vi "CDW_SpecPage.vi"(10 "Spec Page Interface":T2, 11 "MetaDataObj in":refnum<class "MetaDataObj.lvclass">) -> (3 "MetaDataObj out":refnum<class "MetaDataObj.lvclass">)   [LabVIEW 2023, in "NIVS_Consolidated_CDW_MetaDataObj.lvclass"]
uses:
  NIVS_Consolidated_CDW_MetaDataObj.lvclass
  <resource>/dialog/NewProjectWizard/Spec Page Interface.ctl
  <resource>/dialog/NewProjectWizard/MetaDataObj/MetaDataObj.lvclass
  C:/Program Files/National Instruments/LabVIEW 2024/resource/dialog/NewProjectWizard/MetaDataObj/MetaDataObj.lvclass
  Template Classes/NIVS_Asynchronous/NIVS_Asynchronous.lvclass
  C:/dev/Karthick/FPGA Addons Packages/niveristand-custom-device-wizard/ProjectTemplate/Source/NI VeriStand/Custom Device/Template Classes/NIVS_CD Template/NIVS_CD Template.lvclass
  Template Classes/NIVS_Inline HW Interface (Inline-Async)/NIVS_Inline HW Interface (Inline-Async).lvclass
  Template Classes/NIVS_Inline HW Interface/NIVS_Inline HW Interface.lvclass
  Template Classes/NIVS_PPL_Inline HW Interface (Inline-Async)/NIVS_PPL_Inline HW Interface (Inline-Async).lvclass
  C:/dev/Karthick/FPGA Addons Packages/niveristand-custom-device-wizard/ProjectTemplate/Source/NI VeriStand/Custom Device/Template Classes/NIVS_PPLCD Template/NIVS_PPLCD Template.lvclass
  Template Classes/NIVS_PPL_Inline HW Interface/NIVS_PPL_Inline HW Interface.lvclass
  Template Classes/NIVS_Inline Model Interface/NIVS_Inline Model Interface.lvclass
  Template Classes/NIVS_Inline Timing and Sync/NIVS_Inline Timing and Sync.lvclass
  Template Classes/NIVS_Asynchronous Timing and Sync/NIVS_Asynchronous Timing and Sync.lvclass
  Template Classes/NIVS_CD Template/NIVS_CD Template.lvclass/NIVS_CD Template.ctl
  NIVS_Consolidated_CDW_MetaDataObj.lvclass/NIVS_Consolidated_CDW_MetaDataObj.ctl
  <resource>/dialog/NewProjectWizard/MetaDataObj/MetaDataObj.lvclass/MetaDataObj.ctl
  Execution Mode.ctl
  Template Classes/NIVS_CD Template/Write Max Instances.vi
  Template Classes/NIVS_CD Template/Write Extra Page Names.vi
  Template Classes/NIVS_CD Template/Write Submenu.vi
  Template Classes/NIVS_CD Template/Write Parent Menu.vi
  Template Classes/NIVS_CD Template/Write Support Runtime Configuration.vi
  <resource>/dialog/NewProjectWizard/MetaDataObj/Accessors/Write Project Name.vi
  <resource>/dialog/NewProjectWizard/MetaDataObj/Accessors/Write Project Root.vi
  Template Classes/NIVS_PPLCD Template/NIVS_PPLCD Template.lvclass
  Template Classes/NIVS_CD Template/NIVS_CD Template.lvclass
panel:
  in  "PPL Build":bool
  in  "Inline-Async":bool=TRUE
  in  "Custom Device Execution Mode":T1(ring)=enum."Inline HW Interface"
  in  "Custom Device Name":string
  in  "Project Root":path
  in  "Support Runtime Configuration":bool
  in  "Maximum Custom Device Instances":i32=1 min=-1 max=2474 step=1
  in  "Insert Custom Device in submenu":bool
  in  "Parent Menu Name":string
  in  "Custom Device Extra Page Names":string[](array[string])
  # "Advanced Options"
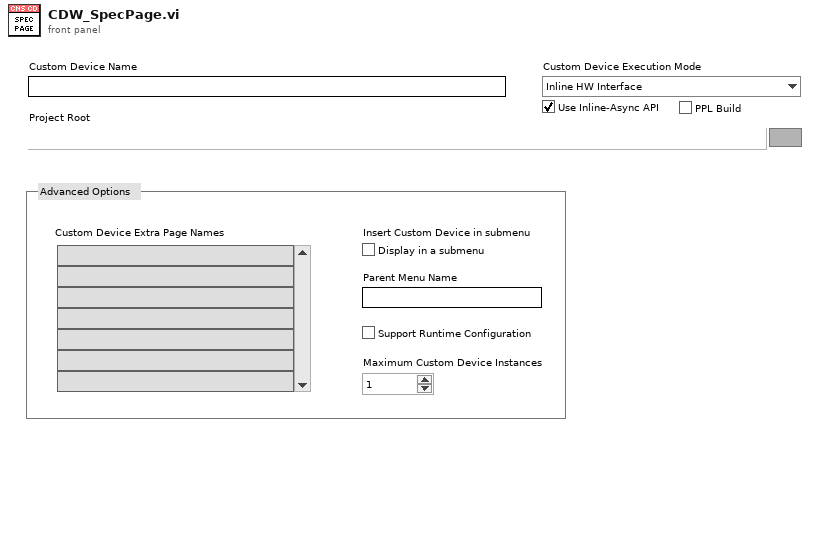
[diagram p1: front panel]
types:
  T1 = enum16{"Asynchronous", "Inline HW Interface", "Inline Model Interface", "Inline Timing and Sync", "Asynchronous Timing and Sync"}
  T2 = typedef "Spec Page Interface.ctl" = cluster{"\"Tab Forward To\" Refnum":refnum<vi>, "\"Tab Backward To\" Refnum":refnum<vi>, "Errors":refnum<user-event>, "Quit":refnum<user-event>}
  T3 = enum8{"Enabled", "Disabled", "Disabled and Grayed Out"}
  T4 = typedef "NIVS_Consolidated_CDW_MetaDataObj.lvclass/Execution Mode.ctl" = enum16{"Asynchronous", "Inline HW Interface", "Inline Model Interface", "Inline Timing and Sync", "Asynchronous Timing and Sync"}
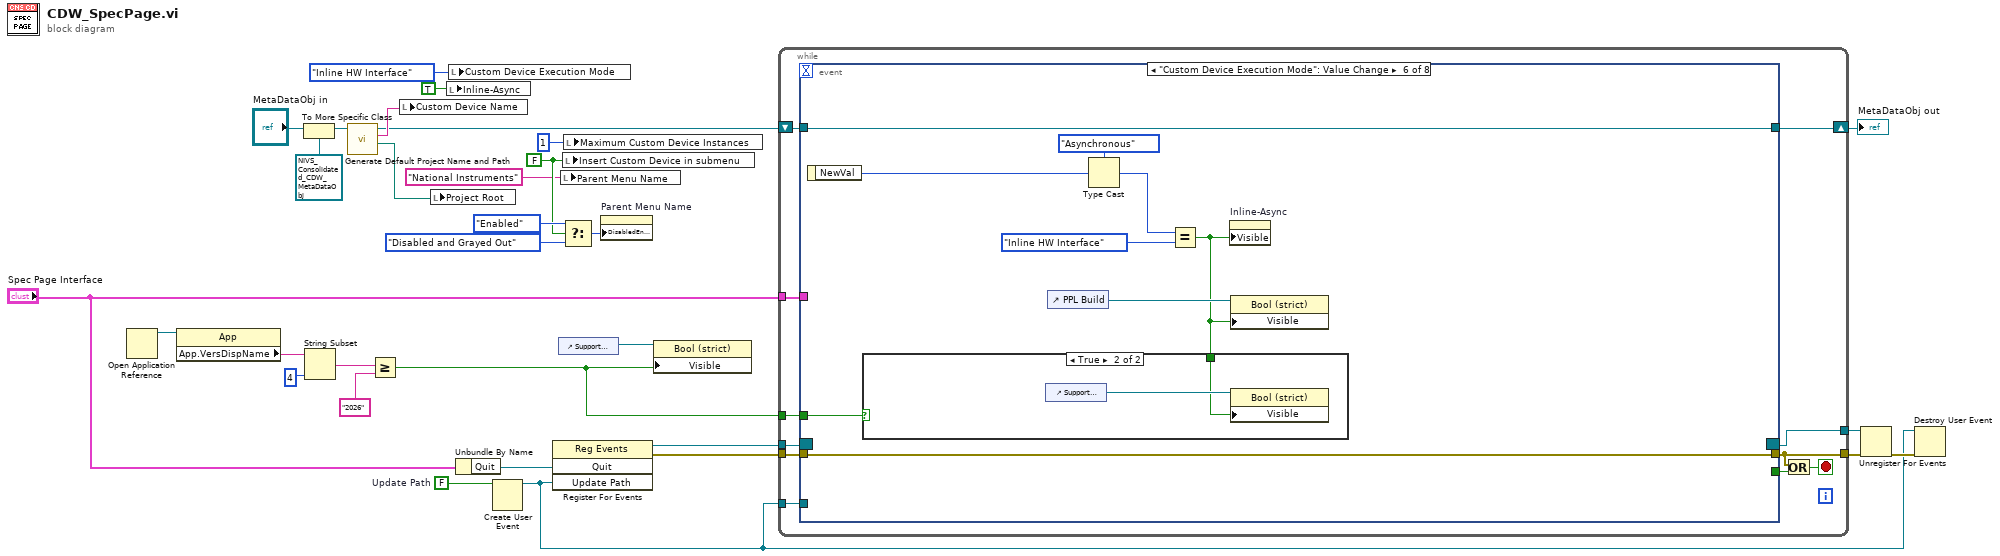
[diagram p0: block diagram]
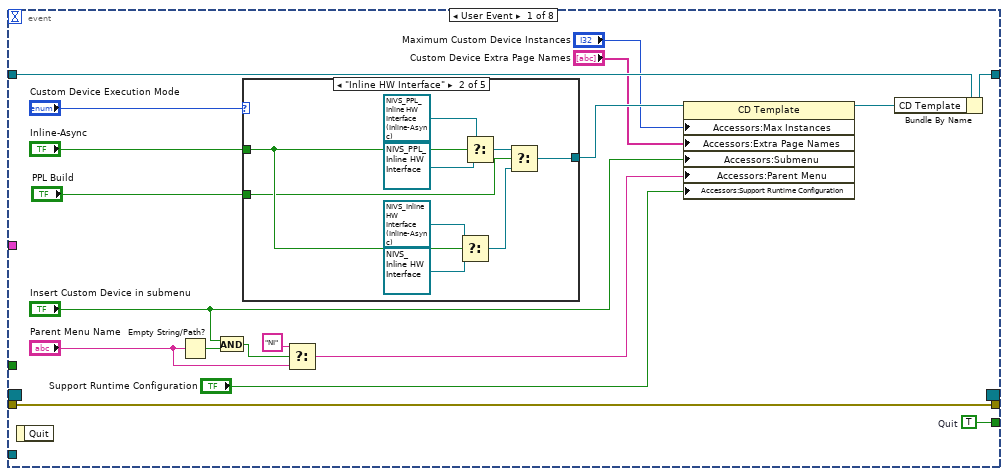
[diagram p2: hidden frame]
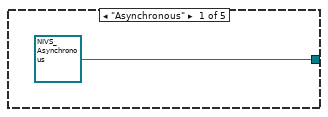
[diagram p3: hidden frame]
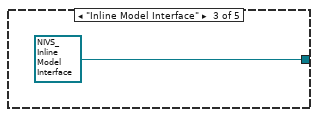
[diagram p4: hidden frame]
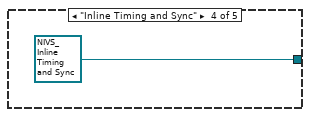
[diagram p5: hidden frame]
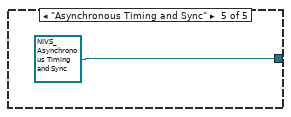
[diagram p6: hidden frame]
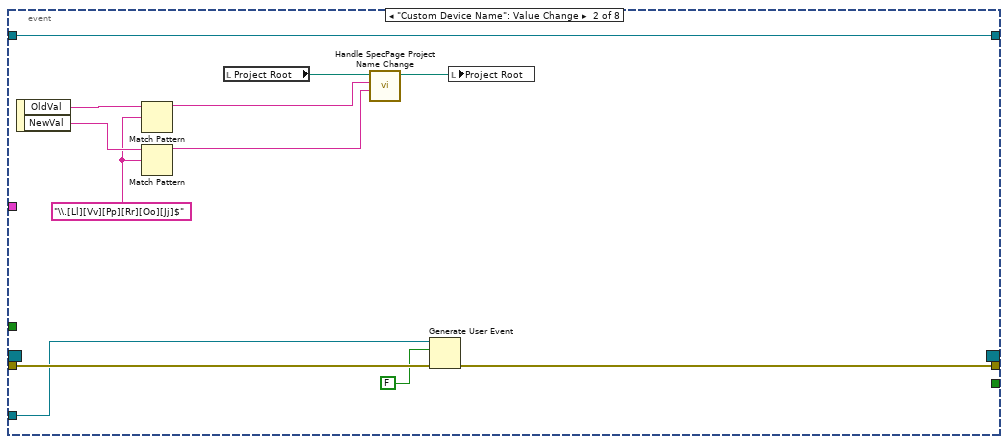
[diagram p7: hidden frame]
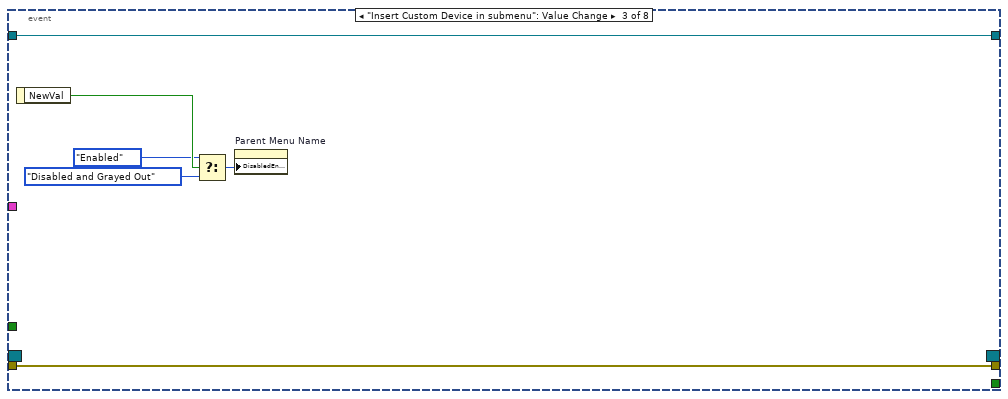
[diagram p8: hidden frame]
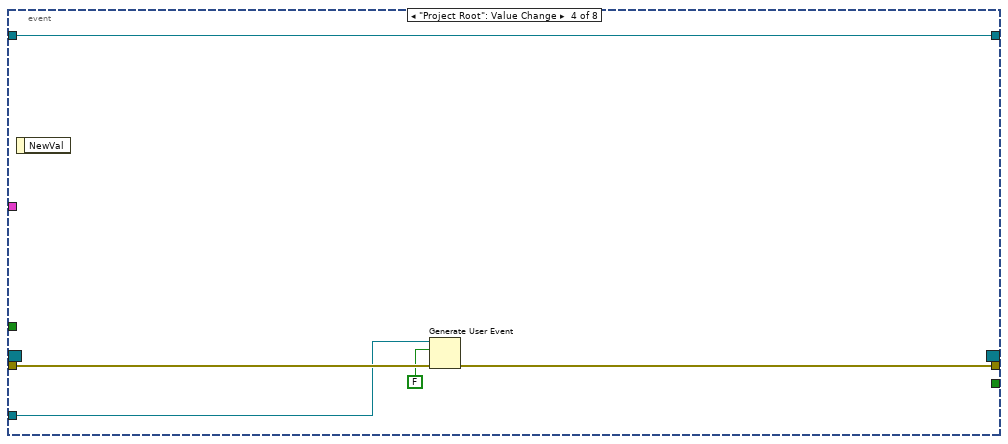
[diagram p9: hidden frame]
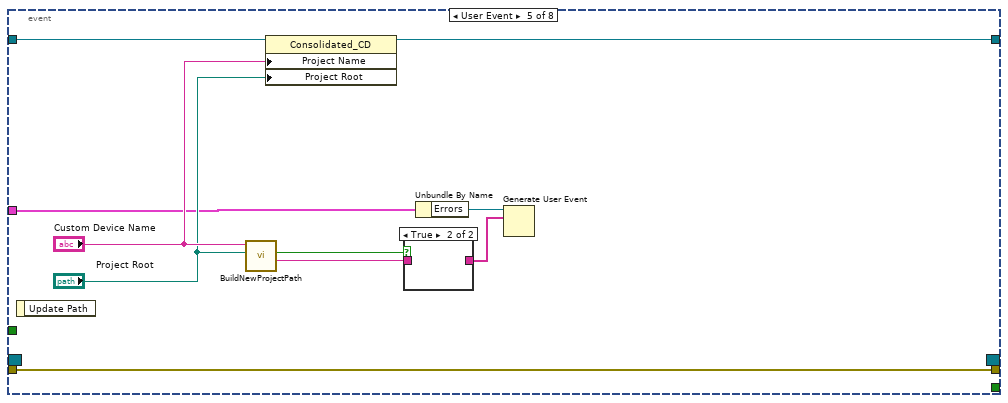
[diagram p10: hidden frame]
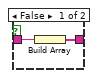
[diagram p11: hidden frame]
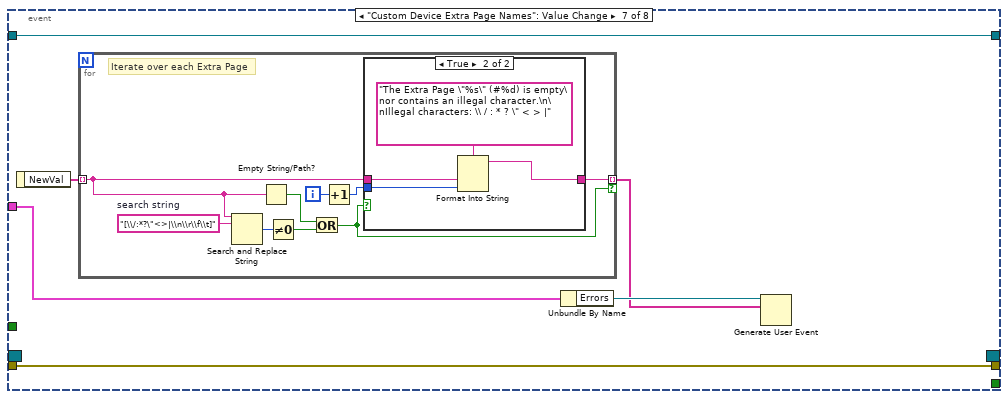
[diagram p13: hidden frame]
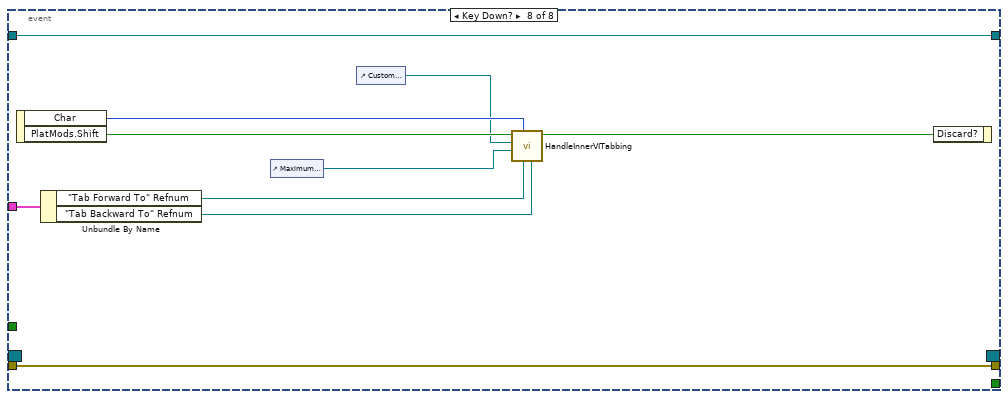
[diagram p15: hidden frame]
diagram:
  w12 = FALSE
  w15 = FALSE  # Update Path
  n1 = Open Application Reference() -> (3:w7:refnum<vi>)  [unwired: 4 in, 1 out]
  n2 = property class="App"(reference=w7) -> ("App.VersDispName"=w6:string)  [unwired: 1 in, 2 out]
  n3 = To More Specific Class(target class=refnum<class "NIVS_Consolidated_CDW_MetaDataObj.lvclass"> refnum ("Consolidated"), reference="MetaDataObj in") -> (specific class reference=w18:refnum<class "NIVS_Consolidated_CDW_MetaDataObj.lvclass">)  [unwired: 1 in, 1 out]
  n4 = String Subset(string=w6, length (rest)=4 ("length (rest)")) -> (substring=w5:string)  [unwired: 1 in]
  n5 = call <resource>:"Generate Default Project Name and Path.vi"("DNL_MetaDataObj in"=w18) -> ("Project Root"=w16:path, "Project Name"=w21:string, "DNL_MetaDataObj out"=w17:refnum<class "NIVS_Consolidated_CDW_MetaDataObj.lvclass">)  [unwired: 8 in]
  n6 = Greater Or Equal?(x=w5, y="2026") -> (x >= y?=w1:bool)
  n7 = local write "Custom Device Name"(w21) -> ()
  n8 = local write "Project Root"(w16) -> ()
  n9 = local write "Inline-Async"(TRUE ("Inline-Async")) -> ()
  n10 = local write "Custom Device Execution Mode"(T1."Inline HW Interface" ("Custom Device Execution Mode")) -> ()
  n11 = Unbundle By Name("Spec Page Interface") -> ("Quit"=w31:refnum<user-event>)
  n12 = Create User Event(user event datatype=w15) -> (user event=w13:refnum<user-event>)  [unwired: 1 in, 1 out]
  n13 = register-events(w31, w13) -> (reference out=w30:refnum<event-registration>, error out=w26:errorcluster)  [unwired: 2 in]
  n14 = control-ref of="Support Runtime Configuration"() -> (w2:refnum<vi>)
  n15 = local write "Parent Menu Name"("National Instruments") -> ()
  n16 = local write "Insert Custom Device in submenu"(w12) -> ()
  n17 = Select(t=T3."Enabled" ("Disabled"), s=w12, f=T3."Disabled and Grayed Out") -> (s? t:f=w24:T3)
  n18 = local write "Maximum Custom Device Instances"(u32 1 ("Maximum Custom Device Instances")) -> ()
  n19 = property on="Parent Menu Name" class="Str"("DisabledEnum"=w24) -> ()  [unwired: 2 in, 2 out]
  n20 = property class="Bool (strict)"(reference=w2, "Visible"=w1) -> ()  [unwired: 1 in, 2 out]
  n21 = while {
    tunnel: "Spec Page Interface" -> [w40]
    shift-right: [w39] -> w27
    shift-left: w17 -> [w38]
    tunnel: w30 -> [w42]
    tunnel: w26 -> [w41]
    tunnel: [w35] -> w28
    tunnel: [w34] -> w20
    tunnel: w13 -> [w33]
    tunnel: w1 -> [w32]
    stop <- w37 stop-if-true
    n22 = event shown="[5] \"Custom Device Execution Mode\": Value Change" {
      selector: w42 -> [_ _ _ _ _ _ _ _]
      dyn-events: [_ _ _ _ _ _ _ _] -> w34
      timeout: _ -> [_ _ _ _ _ _ _ _]
      tunnel: w40 -> [_ _ _ _ w101 _ w121 w144]
      tunnel: [w60 _ _ _ _ _ _ _] -> w36
      tunnel: [w59 w76 w91 w94 w106 w117 w125 w149] -> w35
      tunnel: w41 -> [w59 w85 w91 w96 w106 w117 w125 w149]
      tunnel: [w57 w84 w90 w95 w104 w116 w123 w148] -> w39
      tunnel: w38 -> [w58 w84 w90 w95 w105 w116 w123 w148]
      tunnel: w33 -> [_ w75 _ w93 _ _ _ _]
      tunnel: w32 -> [_ _ _ _ _ w109 _ _]
      event User Event {
        w60 = TRUE  # Quit
        n23 = event-data() -> ()  [unwired: 1 in, 1 out]
        n24 = Empty String/Path?(string/path="Parent Menu Name") -> (empty?=w55:bool)
        n25 = And(x="Insert Custom Device in submenu", y=w55) -> (x .and. y?=w54:bool)
        n26 = case shown="\"Inline HW Interface\"" "Custom Device Execution Mode" {
          tunnel: "Inline-Async" -> [_ w63 _ _ _]
          tunnel: [refnum<class "NIVS_Asynchronous.lvclass"> refnum ("NIVS_Asynchronous.lvclass") w65 refnum<class "NIVS_Inline Model Interface.lvclass"> refnum ("NIVS_Inline Model Interface.lvclass") refnum<class "NIVS_Inline Timing and Sync.lvclass"> refnum ("NIVS_Inline Timing and Sync.lvclass") refnum<class "NIVS_Asynchronous Timing and Sync.lvclass"> refnum ("NIVS_Asynchronous Timing and Sync.lvclass")] -> w49
          tunnel: "PPL Build" -> [_ w62 _ _ _]
          frame "Asynchronous" {
          }
          frame "Inline HW Interface" {
            n27 = Select(t=refnum<class "NIVS_Inline HW Interface (Inline-Async).lvclass"> refnum ("NIVS_Inline HW Interface (Inline-Async).lvclass"), s=w63, f=refnum<class "NIVS_Inline HW Interface.lvclass"> refnum ("NIVS_Inline HW Interface.lvclass")) -> (s? t:f=w64:refnum<class "NIVS_CD Template.lvclass">)
            n28 = Select(t=refnum<class "NIVS_PPL_Inline HW Interface (Inline-Async).lvclass"> refnum ("NIVS_PPL_Inline HW Interface (Inline-Async).lvclass"), s=w63, f=refnum<class "NIVS_PPL_Inline HW Interface.lvclass"> refnum ("NIVS_PPL_Inline HW Interface.lvclass")) -> (s? t:f=w66:refnum<class "NIVS_PPLCD Template.lvclass">)
            n29 = Select(t=w66, s=w62, f=w64) -> (s? t:f=w65:refnum<class "NIVS_CD Template.lvclass">)
          }
          frame "Inline Model Interface" {
          }
          frame "Inline Timing and Sync" {
          }
          frame "Asynchronous Timing and Sync" {
          }
        }
        n30 = Select(t="NI", s=w54, f="Parent Menu Name") -> (s? t:f=w45:string)
        n31 = property class="CD Template"(reference=w49, "Accessors:Max Instances"="Maximum Custom Device Instances", "Accessors:Extra Page Names"="Custom Device Extra Page Names", "Accessors:Submenu"="Insert Custom Device in submenu", "Accessors:Parent Menu"=w45, "Accessors:Support Runtime Configuration"="Support Runtime Configuration") -> (reference out=w50:refnum<class "NIVS_CD Template.lvclass">)  [unwired: 1 in, 1 out]
        n32 = Bundle By Name(cluster=w58, "CD Template"=w50) -> (w57:refnum<class "NIVS_Consolidated_CDW_MetaDataObj.lvclass">)
      }
      event "Custom Device Name": Value Change {
        w81 = "\\.[Ll][Vv][Pp][Rr][Oo][Jj]$"
        n33 = event-data() -> ("OldVal"=w83:string, "NewVal"=w82:string)  [unwired: 1 in]
        n34 = Match Pattern(string=w83, regular expression=w81) -> (before substring=w78:string)  [unwired: 1 in, 3 out]
        n35 = Match Pattern(string=w82, regular expression=w81) -> (before substring=w77:string)  [unwired: 1 in, 3 out]
        n36 = local read "Project Root"() -> (w80:path)
        n37 = call <resource>:"Handle SpecPage Project Name Change.vi"("Project Name New Value"=w77, "Project Name Old Value"=w78, "Project Root in"=w80) -> ("Project Root out"=w79:path)  [unwired: 8 in]
        n38 = Generate User Event(user event=w75, event data cluster=FALSE, error in=w85) -> (error out=w76:errorcluster)  [unwired: 1 in, 1 out]
        n39 = local write "Project Root"(w79) -> ()
      }
      event "Insert Custom Device in submenu": Value Change {
        n40 = event-data() -> ("NewVal"=w89:bool)  [unwired: 1 in]
        n41 = Select(t=T3."Enabled" ("Disabled"), s=w89, f=T3."Disabled and Grayed Out") -> (s? t:f=w86:T3)
        n42 = property on="Parent Menu Name" class="Str"("DisabledEnum"=w86) -> ()  [unwired: 2 in, 2 out]
      }
      event "Project Root": Value Change {
        n43 = event-data() -> ()  [unwired: 1 in, 1 out]
        n44 = Generate User Event(user event=w93, event data cluster=FALSE, error in=w96) -> (error out=w94:errorcluster)  [unwired: 1 in, 1 out]
      }
      event User Event {
        n45 = event-data() -> ()  [unwired: 1 in, 1 out]
        n46 = call <resource>:"BuildNewProjectPath.vi"("Project Root"="Project Root", "Project Name"="Custom Device Name") -> ("Error Message"=w100:string, "Valid?"=w97:bool)  [unwired: 7 in, 1 out]
        n47 = property class="Consolidated_CD"(reference=w105, "Project Name"="Custom Device Name", "Project Root"="Project Root") -> (reference out=w104:refnum<class "NIVS_Consolidated_CDW_MetaDataObj.lvclass">)  [unwired: 1 in, 1 out]
        n48 = case shown="True" w97 {
          tunnel: w100 -> [w108 _]
          tunnel: [w107 _] -> w98
          frame False {
            n49 = Build Array(w108) -> (w107:string[])
          }
          frame True {
          }
        }
        n50 = Unbundle By Name(w101) -> ("Errors"=w99:refnum<user-event>)
        n51 = Generate User Event(user event=w99, event data cluster=w98) -> ()  [unwired: 2 in, 2 out]
      }
      event "Custom Device Execution Mode": Value Change {
        n52 = event-data() -> ("NewVal"=w115:T1)  [unwired: 1 in]
        n53 = control-ref of="PPL Build"() -> (w111:refnum<vi>)
        n54 = Type Cast(type=Execution_Mode."Asynchronous" ("CD Wizard - Internal Data.Common Information.CD Execution Mode"), x=w115) -> (*(type *) &x=w113:T4)
        n55 = Equal?(x=w113, y=Execution_Mode."Inline HW Interface") -> (x = y?=w110:bool)
        n56 = case shown="True" w109 {
          tunnel: w110 -> [_ w118]
          frame False {
          }
          frame True {
            n57 = control-ref of="Support Runtime Configuration"() -> (w119:refnum<vi>)
            n58 = property class="Bool (strict)"(reference=w119, "Visible"=w118) -> ()  [unwired: 1 in, 2 out]
          }
        }
        n59 = property on="Inline-Async" class="Bool (strict)"("Visible"=w110) -> ()  [unwired: 2 in, 2 out]
        n60 = property class="Bool (strict)"(reference=w111, "Visible"=w110) -> ()  [unwired: 1 in, 2 out]
      }
      event "Custom Device Extra Page Names": Value Change {
        n61 = event-data() -> ("NewVal"=w124:string[])  [unwired: 1 in]
        n62 = for {
          tunnel: w124 -> [w128] mode=indexing
          tunnel: [w127] -> w120 mode=indexing if=w126
          i -> [w130]
          w134 = "[\\/:*?\"<>|\\n\\r\\f\\t]"  # search string
          # "Iterate over each Extra Page"
          n63 = Search and Replace String(input string=w128, search string=w134) -> (number of replacements=w133:i32)  [unwired: 6 in, 3 out]
          n64 = Empty String/Path?(string/path=w128) -> (empty?=w132:bool)
          n65 = Not Equal To 0?(x=w133) -> (x != 0?=w131:bool)
          n66 = Or(x=w132, y=w131) -> (x .or. y?=w126:bool)
          n67 = Increment(x=w130) -> (x+1=w129:i32)
          n68 = case shown="True" w126 {
            tunnel: w129 -> [_ w137]
            tunnel: w128 -> [w135 w138]
            tunnel: [w135 w136] -> w127
            frame False {
              # "Extra Page Name is OK"
            }
            frame True {
              n69 = Format Into String(format string="The Extra Page \"%s\" (#%d) is empty\nor contains an illegal character.\n\nIllegal characters: \\ / : * ? \" < > |", w138, w137) -> (resulting string=w136:string)  [unwired: 2 in, 1 out]
            }
          }
        }
        n70 = Unbundle By Name(w121) -> ("Errors"=w122:refnum<user-event>)
        n71 = Generate User Event(user event=w122, event data cluster=w120) -> ()  [unwired: 2 in, 2 out]
      }
      event Key Down? {
        n72 = event-data() -> ("Char"=w147:i16, "PlatMods.Shift"=w146:bool)  [unwired: 1 in]
        n73 = Unbundle By Name(w144) -> ("\"Tab Forward To\" Refnum"=w143:refnum<vi>, "\"Tab Backward To\" Refnum"=w142:refnum<vi>)
        n74 = control-ref of="Maximum Custom Device Instances"() -> (w140:refnum<vi>)
        n75 = control-ref of="Custom Device Name"() -> (w141:refnum<vi>)
        n76 = call <resource>:"HandleInnerVITabbing.vi"("Tab Backward To"=w142, "Tab Forward To"=w143, "Char"=w147, "Last Control"=w140, "First Control"=w141, "Shift"=w146) -> ("Discard"=w145:bool)  [unwired: 5 in]
        n77 = event-data("Discard?"=w145) -> ()  [unwired: 1 in, 1 out]
      }
    }
    n78 = Or(x=w35, y=w36) -> (x .or. y?=w37:bool)
  }
  "MetaDataObj out" <- w27
  n79 = Unregister For Events(event registration refnum=w20, error in=w28) -> (error out=w14:errorcluster)
  n80 = Destroy User Event(user event=w13, error in=w14) -> ()  [unwired: 1 out]
